vi "FestoCPX.IO.vi"(8 "error in":errorcluster, 11 "Data in":T1={"Status"={"State"=enum."First", "Conn"=refnum, "TS"=timestamp(0 s since 1904-01-01)}, "Sets"={"IP"="", "Timeout_ms"=1, "ReconnectPeriod_s"=0, "Config.DI"=[], "Config.DO"=[]}}) -> (0 "error out":errorcluster, 3 "Data out":T1={"Status"={"State"=enum."First", "Conn"=refnum, "TS"=timestamp(0 s since 1904-01-01)}, "Sets"={"IP"="", "Timeout_ms"=1, "ReconnectPeriod_s"=0, "Config.DI"=[], "Config.DO"=[]}})   [LabVIEW 2016]
uses:
  FestoCPX.Data.ctl
  FestoCPX.Data.Status.ctl
  FestoCPX.State.ctl
  FestoCPX.Data.Sets.ctl
  FestoCPX.DI.Sets.ctl
  FestoCPX.DI.ctl
  FestoCPX.DO.Sets.ctl
  FestoCPX.DO.ctl
  tools/EventLog/EventLog.EventSource.ctl
panel:
  out "chart":u32(graph)
  out "delay":u32
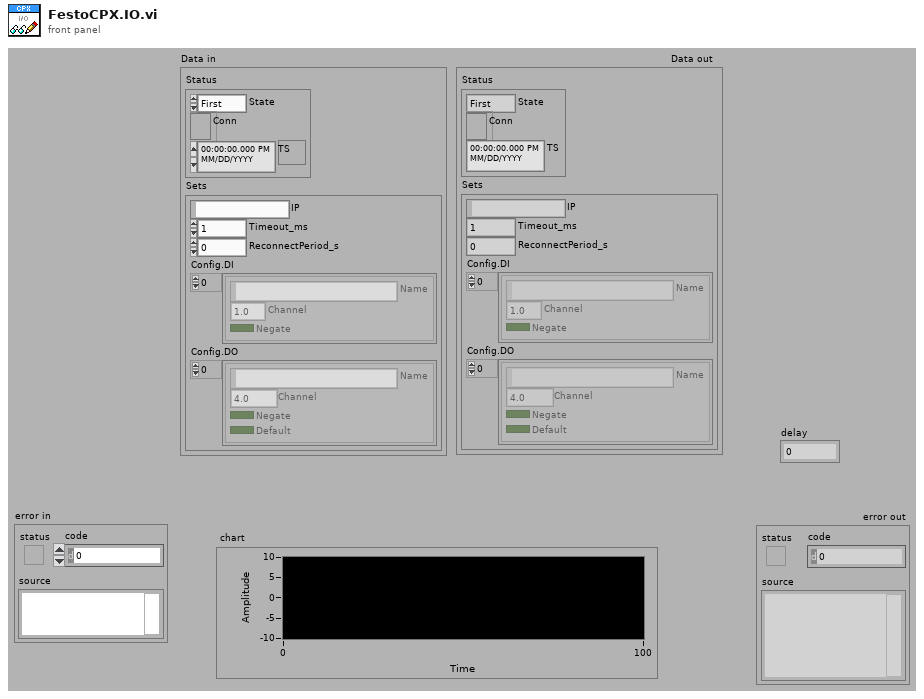
[diagram p1: front panel]
types:
  T1 = typedef "FestoCPX.Data.ctl" = cluster{"Status":T2, "Sets":T4}
  T2 = typedef "FestoCPX.Data.Status.ctl" = cluster{"State":T3, "Conn":refnum<k5>, "TS":timestamp}
  T3 = typedef "FestoCPX.State.ctl" = enum16{"First", "Error", "Init", "Run"}
  T4 = typedef "FestoCPX.Data.Sets.ctl" = cluster{"IP":string, "Timeout_ms":i32, "ReconnectPeriod_s":i32, "Config.DI":T5[], "Config.DO":T7[]}
  T5 = typedef "FestoCPX.DI.Sets.ctl" = cluster{"Name":string, "Channel":T6, "Negate":bool}
  T6 = typedef "FestoCPX.DI.ctl" = enum16{"0.0", "0.1", "0.2", "0.3", "0.4", "0.5", "0.6", "0.7", "1.0", "1.1", "1.2", "1.3", "1.4", "1.5", "1.6", "1.7", "2.0", "2.1", "2.2", "2.3", "2.4", "2.5", "2.6", "2.7", "3.0", "3.1", "3.2", "3.3", "3.4", "3.5", "3.6", "3.7", "4.0", "4.1", "4.2", "4.3", "4.4", "4.5", "4.6", "4.7"}
  T7 = typedef "FestoCPX.DO.Sets.ctl" = cluster{"Name":string, "Channel":T8, "Negate":bool, "Default":bool}
  T8 = typedef "FestoCPX.DO.ctl" = enum16{"4.0", "4.1", "4.2", "4.3", "4.4", "4.5", "4.6", "4.7", "5.0", "5.1", "5.2", "5.3", "5.4", "5.5", "5.6", "5.7", "6.0", "6.1", "6.2", "6.3", "6.4", "6.5", "6.6", "6.7", "Q1K1", "Q1K2", "Q2K1", "Q2K2", "Q3K1", "Q3K2", "Q4K1", "Q4K2", "Q5K1", "Q5K2", "Q6K1", "Q6K2"}
  T9 = typedef "EventLog.EventSource.ctl" = enum16{"All", "Gui", "Ref", "File", "Arch", "Seq", "CPX", "DB", "Laser", "Scan.P", "Scan.O"}
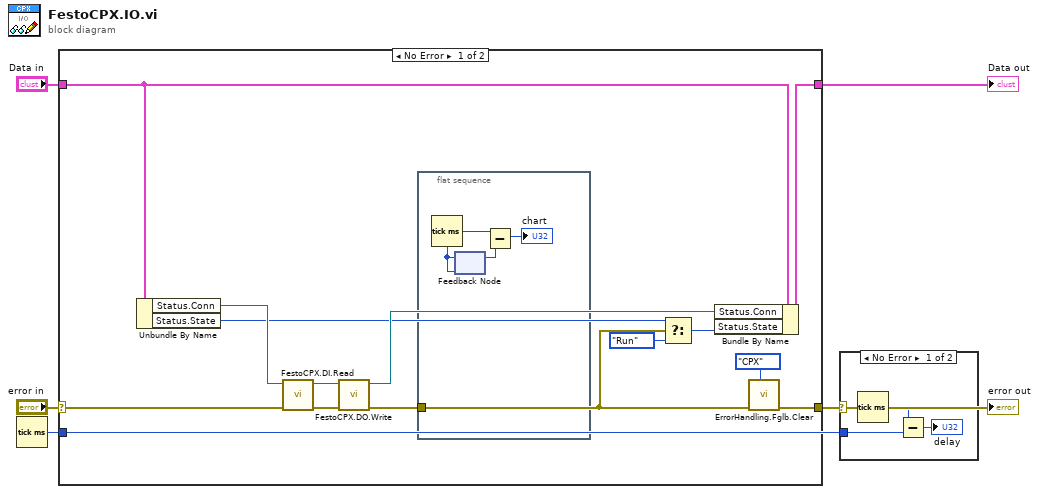
[diagram p0: block diagram]
diagram:
  n1 = Tick Count (ms)() -> (millisecond timer value=w1:u32)
  n2 = case shown="No Error" "error in" {
    selector: "error in" -> [w18 w23]
    tunnel: "Data in" -> [w15 w22]
    tunnel: [w14 w22] -> w4
    tunnel: [w11 w23] -> w2
    tunnel: w1 -> [_ _]
    frame No Error {
      n3 = Unbundle By Name(w15) -> ("Status.Conn"=w8:refnum<k5>, "Status.State"=w7:T3)
      n4 = call "FestoCPX.DI.Read.vi"("error in (no error)"=w18, "TCP Conn Ref"=w8) -> ("error out"=w17:errorcluster, "TCP Conn Ref out"=w16:refnum<k5>)  [unwired: 8 in]
      n5 = call "FestoCPX.DO.Write.vi"("error in (no error)"=w17, "TCP Conn Ref"=w16) -> ("error out"=w6:errorcluster, "TCP Conn Ref out"=w13:refnum<k5>)  [unwired: 7 in, 1 out]
      n6 = flat-sequence {
        tunnel: w6 -> [_]
        frame #0 {
          n7 = Tick Count (ms)() -> (millisecond timer value=w20:u32)
          n8 = feedback-in #1(w20) -> ()
          n9 = feedback #1(w20) -> (w21:u32)
          n10 = Subtract(x=w20, y=w21) -> (x-y=→"chart":u32)
        }
      }
      n11 = Select(t=w7, s=w6, f=FestoCPX.State."Run") -> (s? t:f=w9:T3)
      n12 = Bundle By Name(cluster=w15, "Status.Conn"=w13, "Status.State"=w9) -> (w14:T1)
      n13 = call "ErrorHandling.Fglb.Clear.vi"("Event source"=EventLog.EventSource."CPX", "error in (no error)"=w6) -> ("error out"=w11:errorcluster)  [unwired: 9 in]
    }
    frame Error {
    }
  }
  "error out" <- w2
  "Data out" <- w4
  n14 = case shown="No Error" w2 {
    tunnel: w1 -> [w25 _]
    frame No Error {
      n15 = Tick Count (ms)() -> (millisecond timer value=w26:u32)
      n16 = Subtract(x=w26, y=w25) -> (x-y=→"delay":u32)
    }
    frame Error {
    }
  }
